vi "Big_LED_control.vi"() -> ()   [LabVIEW 2018]
uses:
  <instrlib>/niDCPower/nidcpower.llb/niDCPower Source Mode.ctl
  <instrlib>/niDCPower/nidcpower.llb/niDCPower Output Function.ctl
  AT lib/AmateurStepperMotor.dll
  <instrlib>/niDMM/nidmm.llb/niDMM Function.ctl
  <instrlib>/niDMM/nidmm.llb/niDMM Resolution in Digits.ctl
  <vilib>/Instr/_visa.llb/VISA Configure Serial Port (Instr).vi
  <instrlib>/niDMM/nidmm.llb/niDMM Configure Measurement Digits.vi
panel:
  out "Voltage Char 2":dbl(graph)=0.2558511793613434
  in  "Tab Control 2":enum32{"Шаговик и офир", "Служебная область"}(tab)
  in  "Go To":dbl
  out "Ophir 1 Char":dbl(graph)=0.02
  in  "DecelerationTime, s":dbl=0.3
  in  "AccelerationTime, s":dbl=0.3
  in  "HoldOn":bool
  in  "Ophir 1 units":string(combo)="1000" caption="Units"
  out "Ophir 1 Optical Power":dbl=0.02 caption="Power" format="%#_4g"
  out "Ophir 1 MAX":dbl=0.02 caption="MAX" format="%#_5g"
  in  "Ophir 1 Clear":bool caption="Clear"
  in  "StepMultiplicationFactor":dbl=50.0
  in  "StepDivisor":i32(ring)=8 items=["D1"=1, "D2"=2, "D4"=4, "D8"=8, "D16"=16, "D32"=32]
  in  "Speed":dbl=250.0
  in  "Погнали!":bool
  in  "Стоп GoTo":bool
  out "Готово":bool
  out "Position":dbl=9.995
  in  "Ophir 1 Info":u16(ring)=1 caption="Info" items=["Device : JUNO; s/n:903793", "Head : PD300R-3W   ; s/n:779628"]
  in  "new pos":dbl
  in  "set pos":bool
  in  "wave_lenght":string="600"
  in  "Ophir 1 usb channel":i16 caption="usb channel"
  out "Ophir 1 dup Visa Session":refnum<visa-resource-name>="USB0::0x0BD3::0x0777::NI-VISA-60003::RAW" caption="dup Visa Session"
  in  "Ophir 1 Baud Rate (3:9600)":i16(ring)=3 caption="Baud Rate (3:9600)" items=["300", "1200", "4800", "9600", "19200", "38400"]
  out "Ophir 1 Real Optical Power":dbl=2e-05 format="%.6e"
  in  "Ophir 1 GPIB Address (10)":string="10" caption="GPIB Address (10)"
  in  "Ophir 1 Port Number (default 2)":i16=1 caption="Port Number (default 2)" min=0 max=20
  in  "Ophir 1 Select Communication Protocol":u16(ring) caption="Select Communication Protocol" items=["USB", "RS232", "GPIB"]
  out "Ophir 1 error out":errorcluster caption="error out"
  in  "Ophir 1 error in (no error)":errorcluster caption="error in (no error)"
  in  "Ophir 1 Wait":u32=100 caption="Wait"
  out "IsOpen":bool
  out "Ophir 1 Initialization":bool=TRUE caption="Initialization"
  out "Device Response":string="*\n"
  in  "Tab Control":T1(tab)
  in  "шаговик":refnum<visa-resource-name>="COM8"
  in  "POWER":bool
  in  "Стоп":bool
  in  "Resource Name":refnum<k15>="PXI1Slot2" caption="Источник питания"
  in  "Амперметр":refnum<k15>="PXI1Slot4" caption="NI DMM 1"
  in  "V_MB, V":dbl=6.0 caption="voltage level" min=0.0 max=6.0 format="%_6p"
  in  "curlim_V_MB, A":dbl=0.3 caption="current limit" format="%_6p"
  out "chart_0":dbl(graph)=-0.00013853853853977013 caption="Waveform Chart 5"
  in  "voltlim_I_LED, V":dbl=2.1 caption="current limit" min=0.01 format="%_6p"
  in  "I_LED, A":dbl=0.010000000000000004 caption="voltage level" format="%_6p"
  out "chart_1":dbl(graph)=-0.0002744397184121777 caption="Waveform Chart 5"
  out "Current Char":dbl(graph)=0.0055655837059021
  in  "Arduino":refnum<visa-resource-name>="COM16"
  in  "Сегменты":bool[](array[boolean])=[FALSE, FALSE, FALSE, FALSE, FALSE, FALSE, FALSE, FALSE, FALSE, FALSE, FALSE, FALSE, FALSE, FALSE, FALSE, FALSE, FALSE, FALSE]
  in  "Вольтметр":refnum<k15>="PXI1Slot5" caption="NI DMM 1"
  out "Voltage Char":dbl(graph)=0.2558511793613434
  in  "Промер":bool caption="Промер сегмента"
  in  "NI DMM 1 Voltage Range 4":string(combo)="-1" caption="Range"
  in  "NI DMM 1 units 4":string(combo)="1" caption="Units"
  out "Voltage":dbl=0.2558511793613434 format="%_6g"
  in  "NI DMM 1 Current Range 3":string(combo)="1" caption="Range"
  in  "NI DMM 1 units 3":string(combo)="1000" caption="Units"
  out "Current":dbl format="%_6g"
  out "voltmes_V_MB, V":dbl=-0.00013853853853977013 caption="measurement" format="%_6g"
  out "curmes_V_MB, A":dbl caption="measurement" format="%_6g"
  out "curmes_I_LED, A":dbl=9.117163901385412e-07 caption="measurement" format="%_6g"
  out "voltmes_I_LED, V":dbl caption="measurement" format="%_6g"
  out "Разряд":dbl
  out "+/-":bool
  out "Power off":bool
  in  "Command":string="Cathode"
  in  "Записать":bool
  out "measure output \nfile refnum":refnum<file>
  out "Voltage, V":dbl=0.2558511793613434 caption="Measurement" format="%.5f"
  out "Current, A":dbl=5.5655837059021e-06 caption="Measurement" format="%.5f"
  out "Тип индикатора":string="Cathode"
  out "chart_2":dbl(graph)=0.0007584113885058215
  in  "V_RES, V":dbl caption="voltage level" format="%_6p"
  out "curmes_V_RES, A":dbl caption="measurement" format="%_6g"
  in  "curlim_V_RES, A":dbl=0.1 caption="current limit" min=0.01 format="%_6p"
  in  "measure path":path=path "C:/Users/user/Desktop/МСП/LabVIEW/LED_CONTROL_big_LED_ophir_24.12.24_1/Logs"
  out "Enum":enum16{"Exit", "4", "Промер", "2", "1"}(ring)
  out "№ об-ца":dbl
  out "Темп-ра":dbl
  out "Сегмент":string="n"
  out "voltmes_V_RES, V":dbl=0.0007584113885058215 caption="measurement" format="%_6g"
  in  "current level range":dbl=0.001 format="%#.6p"
  in  "range on/off":bool
  in  "I (np)":bool
  in  "II (Lm)":bool
  in  "III (jk)":bool
  in  "IV (gh)":bool
  in  "I - IV":bool
  # "Шаговик"
  # "Офир"
  # "Шаговик"
  # "Офир"
  # "position - это значение абсолютное"
  # "j"
  # "c"
  # "d"
  # "e"
  # "g"
  # "h"
  # "a"
  # "b"
  # "f"
  # "k"
  # "L"
  # "m"
  # "n"
  # "p"
  # "dp"
  # "all"
  # "1мА-30мА -> 1m\n10мА-1А -> off"
  # "V_MB 5 В\nогрничение 300 м\n\nV_LED 2,1 В\nограничение 200 м"
  # "единицы мА\nrange 1 А"
  # "1. каждый сегмент включаем по отдельности, резистором постраиваем ток до 10 мА\n2. напряжение V_LED при этом не меняется\n3. в такоом положении промеряем сегменты по отдельности\n4. для промера всего индикатора сразу подстраиваем напряжение при неизменном положении резисторов\n5. ток всех индикаторов = ток одного сегмента (10 мА) * число сегментов (15)\n6. добиваемся этого увеличением V_LED"
  # "единицы В\nrange AUTO"
  # "регклировка суммарного тока через индикатор"
  # "24.063\n\n     I          U\n20 мА  1.3 В\n20 мА  1.4 В\n 7 мА   1.15 В"
  # "24.064\n\n     I          U\n10 мА  2 В\n10 мА  2.15 В\n 7 мА   1.9 В"
  # "автоматизировать подбор напряжения по известному максимальному напряжению и току. ОС по току сегмента"
  # "Р1:  +25°C\nР2:  - 60°C\nР3:  +85°C"
  # "24.067 (в работе)"
  # "регулировать ток в зависимости от температуры.\nс ростом температуры растет ток.\nпид-регулятор??"
  # "0. ввести номер образца\n1. включить нужный сегмент\n2. ввести его в поле справа\n3. вести температуру в поле слева\n4. нажать кнопку \"промер сегмента\""
  # "\"опрашивать кнопки не чаще, чем раз в секунду. сейчас кликать можно чаще, они загорятся, но ничего не произойдет\""
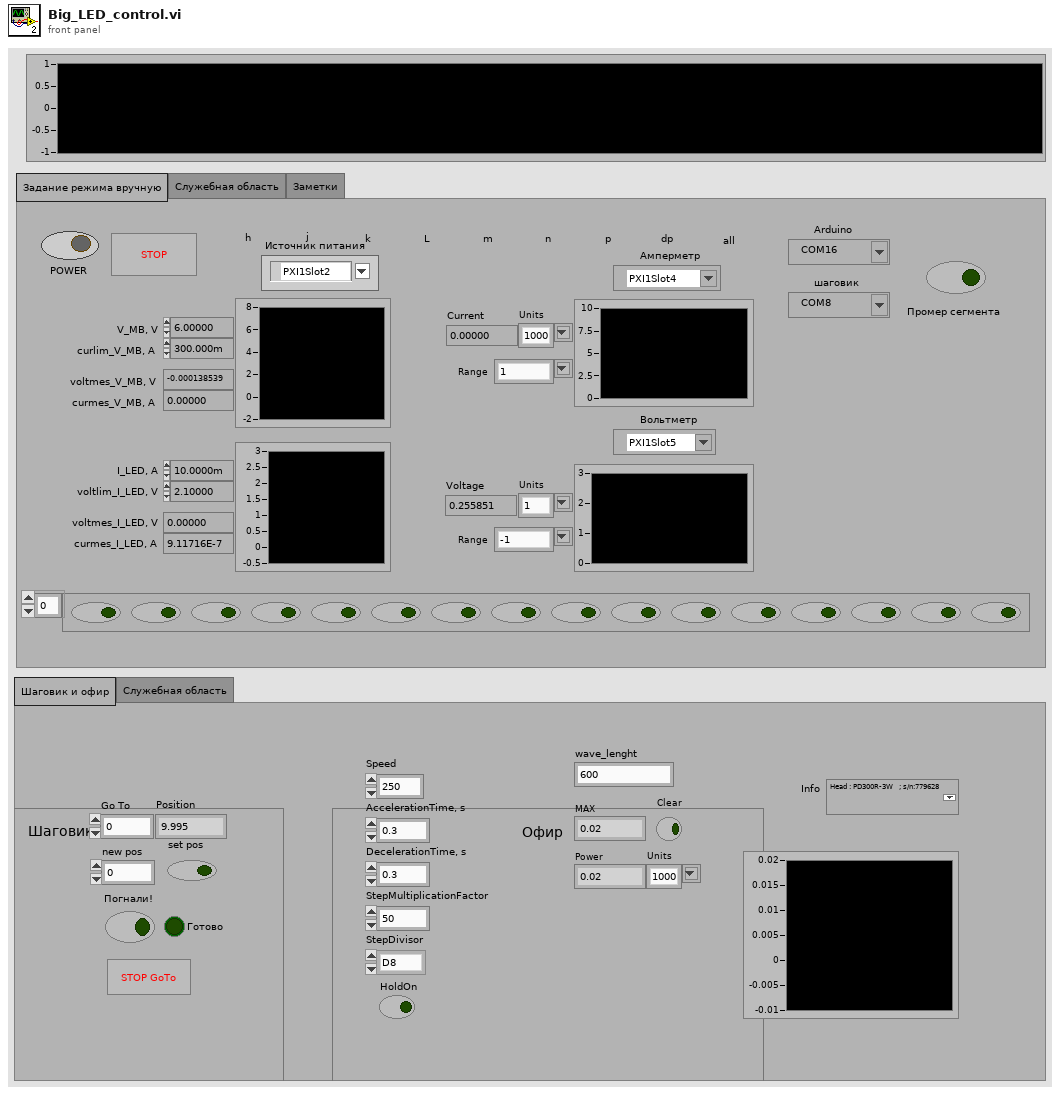
[diagram p1: front panel]
types:
  T1 = enum32{"Задание режима вручную", "Служебная область", "Заметки"}
  T2 = enum16{"open", "replace", "create", "open or create", "replace or create", "replace or create with confirmation"}
  T3 = typedef "niDCPower Output Function.ctl" = i32
  T4 = typedef "niDCPower Source Mode.ctl" = i32
  T5 = typedef "niDMM Function.ctl" = enum16{"DC Volts", "AC Volts", "DC Current", "AC Current", "2-wire Resistance", "4-wire Resistance", "Diode", "Frequency", "Period", "AC Volts DC Coupled", "Capacitance", "Inductance", "Temperature"}
  T6 = typedef "niDMM Resolution in Digits.ctl" = dbl
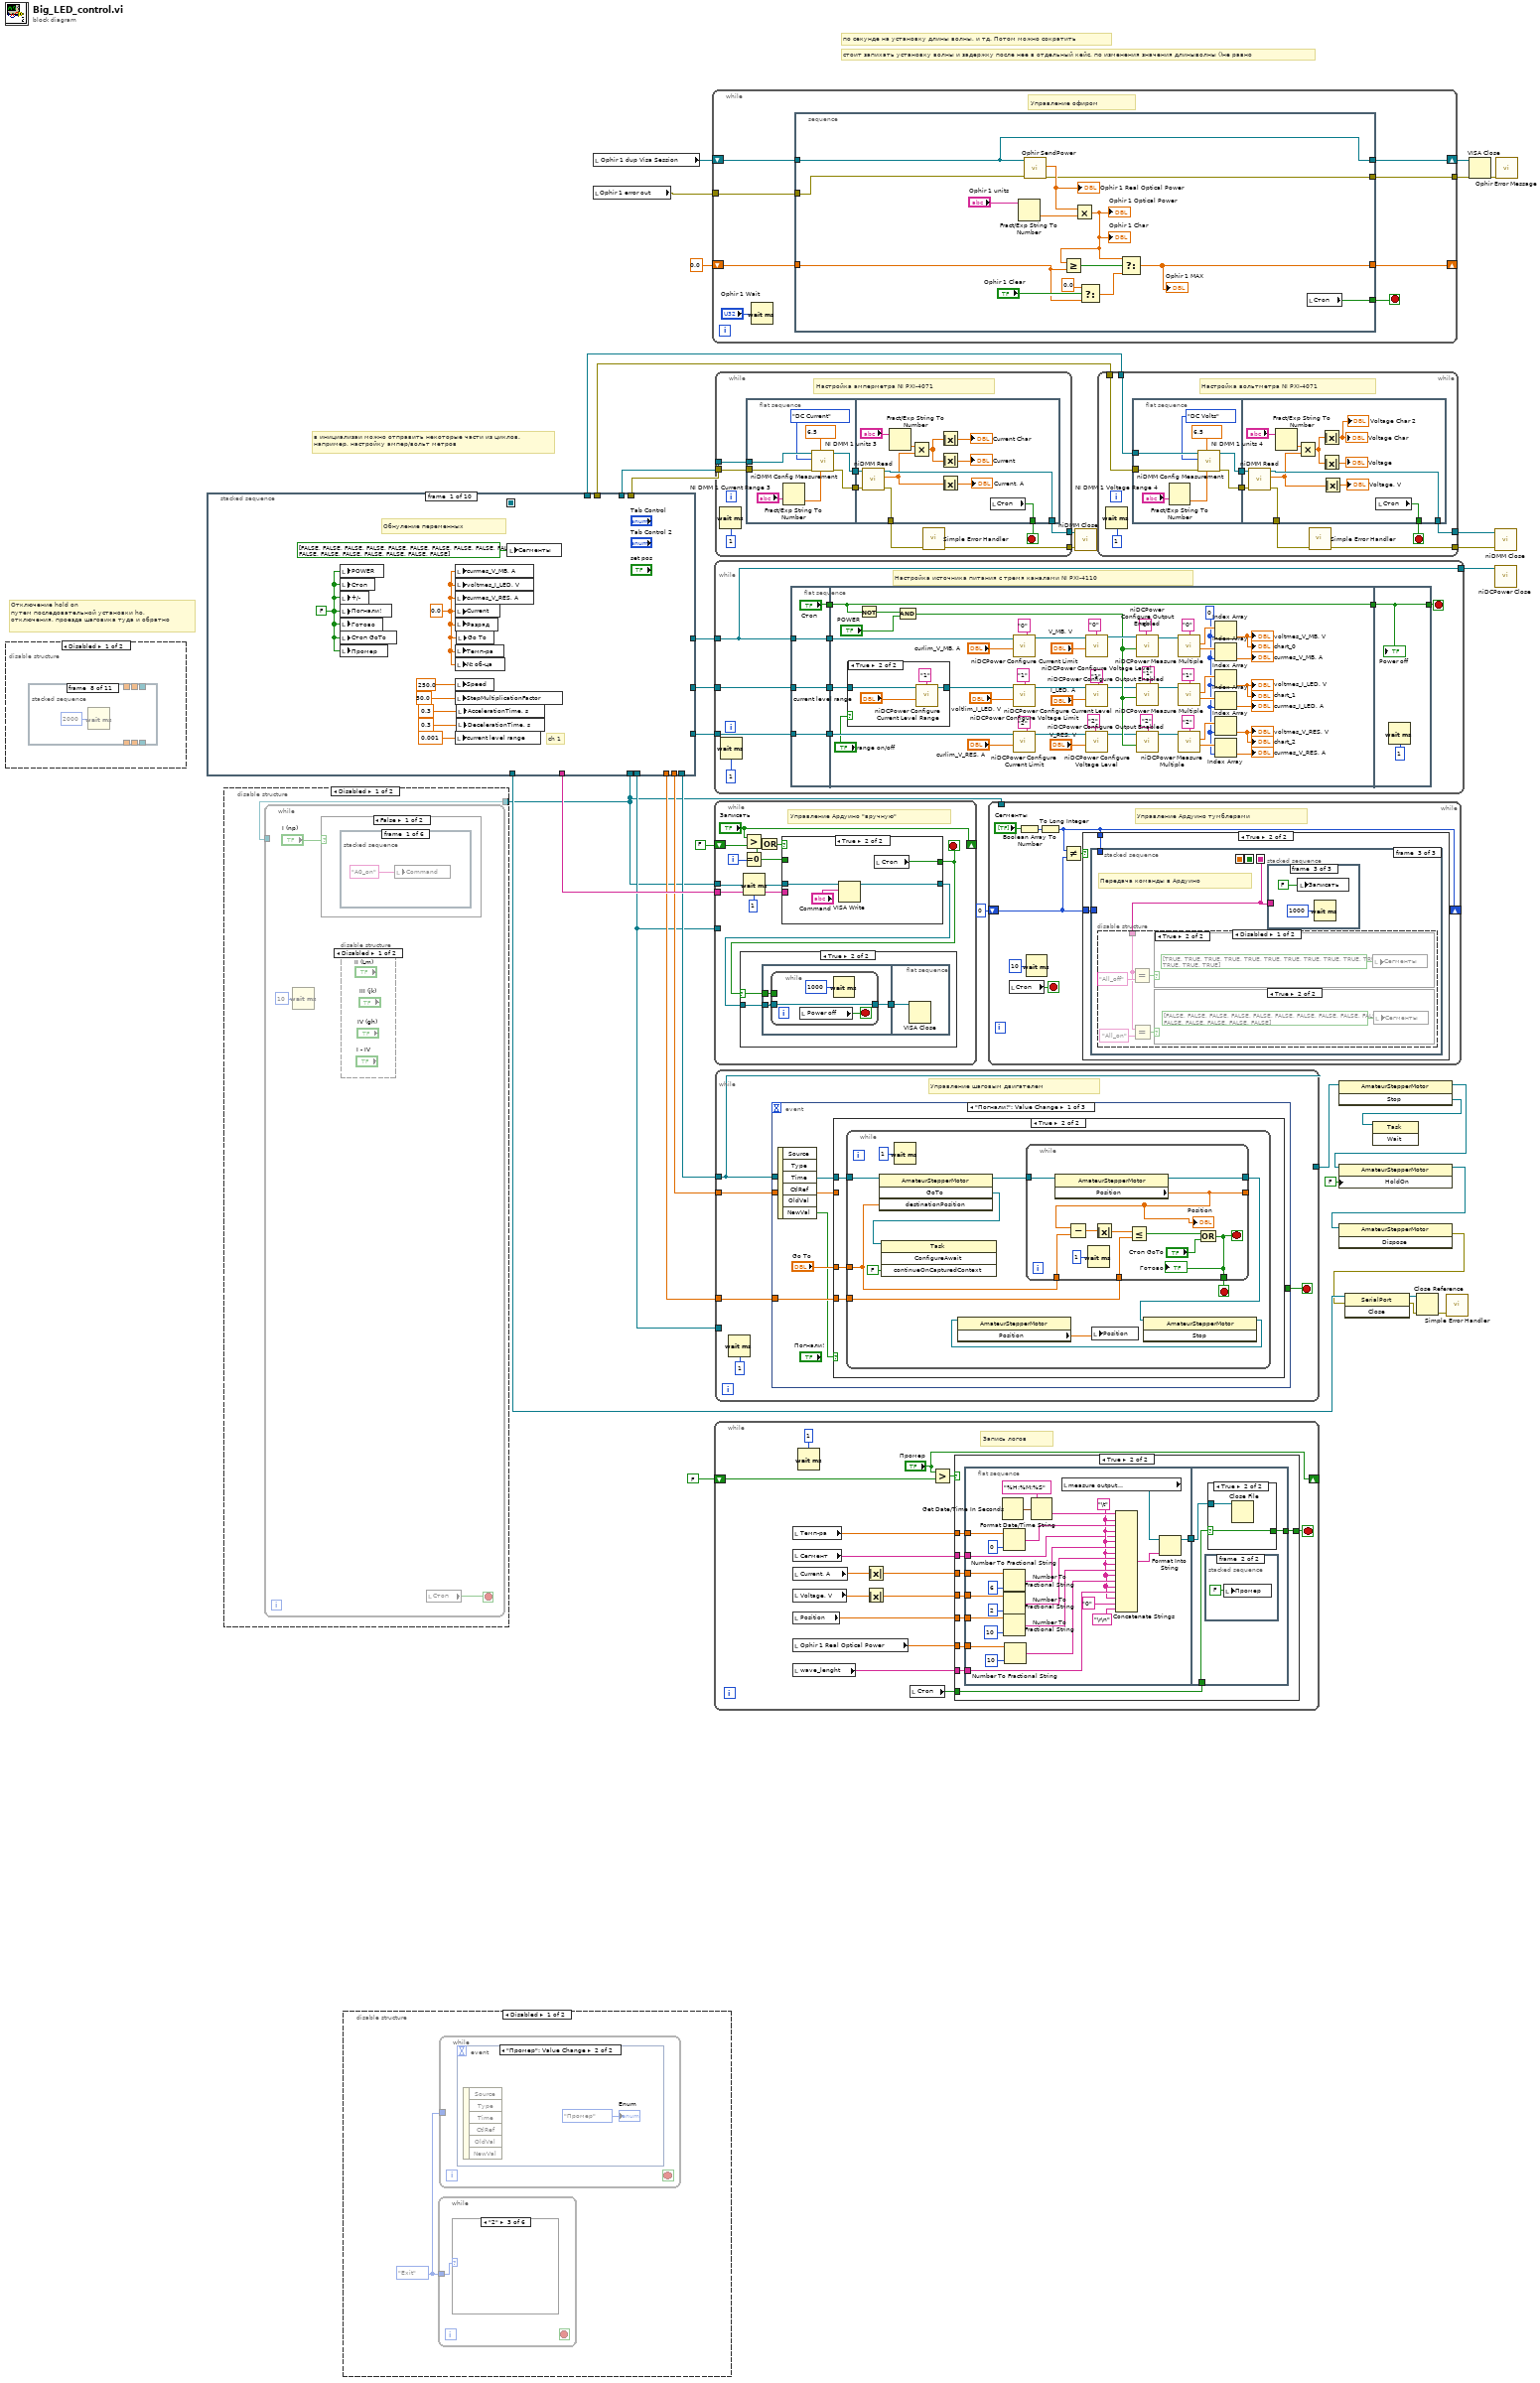
[diagram p0: block diagram]
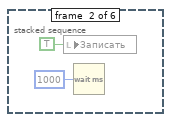
[diagram p3: hidden frame]
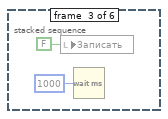
[diagram p4: hidden frame]
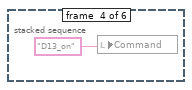
[diagram p5: hidden frame]
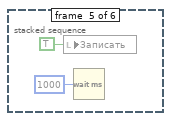
[diagram p6: hidden frame]
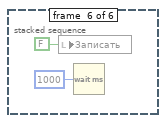
[diagram p7: hidden frame]
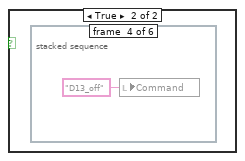
[diagram p8: hidden frame]
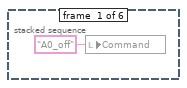
[diagram p9: hidden frame]
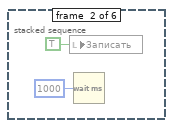
[diagram p10: hidden frame]
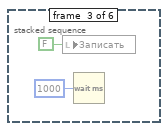
[diagram p11: hidden frame]
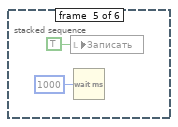
[diagram p12: hidden frame]
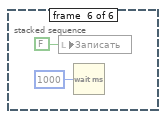
[diagram p13: hidden frame]
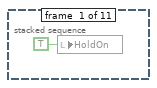
[diagram p15: hidden frame]
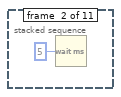
[diagram p16: hidden frame]
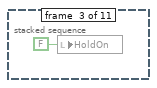
[diagram p17: hidden frame]
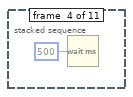
[diagram p18: hidden frame]
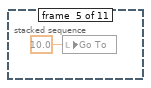
[diagram p19: hidden frame]
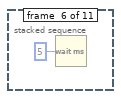
[diagram p20: hidden frame]
diagram:
  # "Отключение hold on\nпутем последовательной установки ho, \nотключения, проезда шаговика туда и обратно"
  # "в инициализаи можно отправить некоторые части из циклов.\nнапример, настройку ампер/вольт метров"
  # "стоит запихать установку волны и задержку после нее в отдельный кейс, по изменения значения длиныволны ()не равно"
  # "по секунде на установку длины волны, и тд. Потом можно сократить"
  n1 = disable-structure shown="Disabled" {
    frame Disabled {
      n2 = stacked-sequence {
        tunnel: _ -> [_ _ _ _ _ _ _ _ _ _ w50]
        tunnel: [_ _ _ _ _ _ _ _ _ _ w50] -> _
        tunnel: _ -> [_ _ _ _ _ _ _ _ _ _ w49]
        tunnel: [_ _ _ _ _ _ _ _ _ _ w49] -> _
        tunnel: [_ _ _ _ _ _ _ _ _ _ w48] -> _
        tunnel: _ -> [_ _ _ _ _ _ _ _ _ _ w48]
        frame #0 {
          n3 = local write "HoldOn"(TRUE ("HoldOn")) -> ()
        }
        frame #1 {
          n4 = Wait (ms)(milliseconds to wait=u32 5) -> ()  [unwired: 1 out]
        }
        frame #2 {
          n5 = local write "HoldOn"(FALSE ("HoldOn")) -> ()
        }
        frame #3 {
          n6 = Wait (ms)(milliseconds to wait=u32 500) -> ()  [unwired: 1 out]
        }
        frame #4 {
          n7 = local write "Go To"(10.0 ("Go To")) -> ()
        }
        frame #5 {
          n8 = Wait (ms)(milliseconds to wait=u32 5) -> ()  [unwired: 1 out]
        }
        frame #6 {
          n9 = local write "Погнали!"(TRUE ("Погнали!")) -> ()
        }
        frame #7 {
          n10 = Wait (ms)(milliseconds to wait=u32 2000) -> ()  [unwired: 1 out]
        }
        frame #8 {
          n11 = local write "Go To"(0.0 ("Go To")) -> ()
        }
        frame #9 {
          n12 = Wait (ms)(milliseconds to wait=u32 5) -> ()  [unwired: 1 out]
        }
        frame #10 {
          n13 = local write "Погнали!"(TRUE ("Погнали!")) -> ()
        }
      }
    }
    frame Enabled {
    }
  }
  n14 = stacked-sequence {
    seq-local: [_ _ _ _ _ _ w117 _ _ _] -> [_ _ _ _ _ _ _ w142 _ _]
    tunnel: [_ _ _ w68 _ _ _ _ _ _] -> w26
    tunnel: [_ w62 _ _ _ _ _ _ _ _] -> w37
    tunnel: [_ w61 _ _ _ _ _ _ _ _] -> w36
    tunnel: [_ _ _ _ w88 _ _ _ _ _] -> w1
    tunnel: [_ _ _ _ _ _ _ _ w148 _] -> w33
    tunnel: [_ _ w65 _ _ _ _ _ _ _] -> w32
    tunnel: [_ _ w64 _ _ _ _ _ _ _] -> w31
    tunnel: [_ _ _ _ _ _ _ w145 _ _] -> w3
    tunnel: [_ _ _ _ _ _ _ w143 _ _] -> w4
    tunnel: [_ _ _ _ _ _ _ w144 _ _] -> w5
    tunnel: [_ _ _ _ _ _ w119 _ _ _] -> w20
    tunnel: [_ _ _ w67 _ _ _ _ _ _] -> w8
    tunnel: [_ _ _ w66 _ _ _ _ _ _] -> w6
    tunnel: [_ _ _ _ _ _ _ _ _ w149] -> w2
    frame #0 {
      w52 = 0.0 ("currentmes_2")
      w53 = FALSE ("Стоп")
      # "ch 1"
      # "Обнуление переменных"
      n15 = local write "POWER"(w53) -> ()
      n16 = local write "Стоп"(w53) -> ()
      n17 = local write "+/-"(w53) -> ()
      n18 = local write "Погнали!"(w53) -> ()
      n19 = local write "Готово"(w53) -> ()
      n20 = local write "Стоп GoTo"(w53) -> ()
      n21 = local write "Промер"(w53) -> ()
      n22 = local write "curmes_V_MB, A"(w52) -> ()
      n23 = local write "voltmes_I_LED, V"(w52) -> ()
      n24 = local write "curmes_V_RES, A"(w52) -> ()
      n25 = local write "Current"(w52) -> ()
      n26 = local write "Разряд"(w52) -> ()
      n27 = local write "Темп-ра"(w52) -> ()
      n28 = local write "№ об-ца"(w52) -> ()
      n29 = local write "Speed"(250.0 ("Speed")) -> ()
      n30 = local write "StepMultiplicationFactor"(50.0 ("StepMultiplicationFactor")) -> ()
      n31 = local write "current level range"(0.001 ("current level range")) -> ()
      n32 = local write "Go To"(w52) -> ()
      n33 = local write "AccelerationTime, s"(0.3 ("AccelerationTime, s")) -> ()
      n34 = local write "DecelerationTime, s"(0.3 ("DecelerationTime, s")) -> ()
      n35 = local write "Сегменты"(bool[] [FALSE, FALSE, FALSE, FALSE, FALSE, FALSE, FALSE, FALSE, FALSE, FALSE, FALSE, FALSE, FALSE, FALSE, FALSE, FALSE, FALSE, FALSE] ("Сегменты")) -> ()
    }
    frame #1 {
      # "Инициализация амперметра"
      n36 = call <instrlib>:"niDMM Initialize.vi"("Instrument Descriptor"="Амперметр") -> ("error out"=w62:errorcluster, "instrument handle out"=w61:refnum<k15>)  [unwired: 9 in]
    }
    frame #2 {
      # "Инициализация вольтметра"
      n37 = call <instrlib>:"niDMM Initialize.vi"("Instrument Descriptor"="Вольтметр") -> ("error out"=w64:errorcluster, "instrument handle out"=w65:refnum<k15>)  [unwired: 9 in]
    }
    frame #3 {
      w73 = T3 1006 items=["DC Voltage"=1006, "DC Current"=1007, "Pulse Voltage"=1049, "Pulse Current"=1050] ("output function")
      w77 = T3 1007 items=["DC Voltage"=1006, "DC Current"=1007, "Pulse Voltage"=1049, "Pulse Current"=1050] ("output function")
      w78 = T3 1006 items=["DC Voltage"=1006, "DC Current"=1007, "Pulse Voltage"=1049, "Pulse Current"=1050] ("output function")
      w81 = T4 1020 items=["Single Point"=1020, "Sequence"=1021] ("source mode")
      # "Инициализация источника питания"
      n38 = call <instrlib>:"niDCPower Initialize.vi"("resource name"="Resource Name") -> ("instrument handle out"=w82:refnum<k15>)  [unwired: 3 in, 7 out]
      n39 = call <instrlib>:"niDCPower Configure Source Mode.vi"("source mode"=w81, "instrument handle"=w82) -> ("instrument handle out"=w72:refnum<k15>)  [unwired: 1 in, 8 out]
      n40 = call <instrlib>:"niDCPower Configure Output Function.vi"("output function"=w77, "channel name"="1", "instrument handle"=w72) -> ("instrument handle out"=w79:refnum<k15>)  [unwired: 7 in, 1 out]
      n41 = call <instrlib>:"niDCPower Configure Output Function.vi"("output function"=w73, "channel name"="2", "instrument handle"=w72) -> ("instrument handle out"=w74:refnum<k15>)  [unwired: 7 in, 1 out]
      n42 = call <instrlib>:"niDCPower Configure Output Function.vi"("output function"=w78, "channel name"="0", "instrument handle"=w72) -> ("instrument handle out"=w80:refnum<k15>)  [unwired: 7 in, 1 out]
      n43 = call <instrlib>:"niDCPower Configure Voltage Level.vi"("voltage level"=0.0, "channel name"="2", "instrument handle"=w74) -> ("instrument handle out"=w66:refnum<k15>)  [unwired: 7 in, 1 out]
      n44 = call <instrlib>:"niDCPower Configure Voltage Level.vi"("voltage level"=0.0, "channel name"="0", "instrument handle"=w80) -> ("instrument handle out"=w68:refnum<k15>)  [unwired: 7 in, 1 out]
      n45 = call <instrlib>:"niDCPower Configure Current Level.vi"("current level"=0.01, "channel name"="1", "instrument handle"=w79) -> ("instrument handle out"=w67:refnum<k15>)  [unwired: 7 in, 1 out]
    }
    frame #4 {
      # "Инициализация Ардуино"
      n46 = call-poly "VISA Configure Serial Port"("VISA resource name"="Arduino", "baud rate (9600)"=u32 9600) -> ("VISA resource name out"=w88:refnum<visa-resource-name>)  [unwired: 12 in, 1 out]
    }
    frame #5 {
      # "Инициализация офира"
      n47 = stacked-sequence {
        frame #0 {
          n48 = call "Ophir InitCom.vi"("GPIB Address (default 10)"="Ophir 1 GPIB Address (10)", "Communication (default USB 0)"="Ophir 1 Select Communication Protocol", "USB Channel number (default 0)"="Ophir 1 usb channel", "Port Number (default 2)"="Ophir 1 Port Number (default 2)", "error in (no error)"="Ophir 1 error in (no error)", "Baud Rate (3:9600)"="Ophir 1 Baud Rate (3:9600)") -> ("dup Visa Session"=w97:refnum<visa-resource-name>, "error out"=w96:errorcluster)  [unwired: 1 out]
          n49 = call "Ophir InstrInfo.vi"("Visa Session"=w97, "error in (no error)"=w96) -> ("dup Visa Session"=w109:refnum<visa-resource-name>, "Instrument Info"=w91:string, "error out"=w107:errorcluster)
          n50 = call "Ophir HeadInfo.vi"("Visa Session"=w109, "error in (no error)"=w107) -> ("error out"=w106:errorcluster, "dup Visa Session"=w108:refnum<visa-resource-name>, "Head Info"=w105:string)  [unwired: 6 out]
          n51 = call "Ophir InfoStrings.vi"("error in (no error)"=w106, "Head Info"=w105, "Instrument Info"=w91) -> ("error out"=w104:errorcluster, "Strings Array"=w103:string[])
          n52 = property on="Ophir 1 Info" class="Ring (strict)"("Strings []"=w103) -> ()  [unwired: 2 in, 2 out]
          n53 = call "Ophir ConfigDevice.vi"("Visa Session"=w108, "Measure Choice (0:Power)"=u16 0, "error in (no error)"=w104) -> ("dup Visa Session"=→"Ophir 1 dup Visa Session":refnum<visa-resource-name>, "OK ?"=→"Ophir 1 Initialization":bool, "error out"=→"Ophir 1 error out":errorcluster)  [unwired: 1 out]
        }
        frame #1 {
          n54 = local read "Ophir 1 dup Visa Session"() -> (w111:refnum<visa-resource-name>)
          n55 = local read "Ophir 1 error out"() -> (w112:errorcluster)
          n56 = call "light_setWaveLenght.vi"("error in (no error)"=w112, "Visa Session"=w111, "wave_lenght"="wave_lenght") -> ("Device Response"=→"Device Response":string)  [unwired: 6 in, 2 out]
        }
      }
    }
    frame #6 {
      w124 = 100 ("WriteTimeout")
      w128 = 1 items=["None", "One", "Two", "OnePointFive"] ("stopBits")
      w126 = 0 items=["None", "Odd", "Even", "Mark", "Space"] ("parity")
      # "убрали открытие порта. шаговик его и так сам откроет"
      # "Инициализация шаговика ч.1"
      n57 = constructor class="SerialPort"("portName"="шаговик", "baudRate"=57600, "parity"=w126, "dataBits"=8, "stopBits"=w128) -> (reference out=w123:refnum<k24>, error out=w122:errorcluster)  [unwired: 3 in, 6 out]
      n58 = property class="SerialPort"(reference=w123, error in=w122, "WriteTimeout"=w124, "ReadTimeout"=w124) -> (reference out=w119:refnum<k24>)  [unwired: 1 out]
      n59 = flat-sequence {
        tunnel: w119 -> [w135]
        tunnel: w118 -> [_]
        frame #0 {
          n60 = property class="SerialPort"(reference=w135) -> ("IsOpen"=→"IsOpen":bool)  [unwired: 1 in, 2 out]
        }
      }
      n61 = constructor class="AmateurStepperMotor"("serialPort"=w119) -> (reference out=w116:refnum<k24>, error out=w115:errorcluster)  [unwired: 3 in, 2 out]
      n62 = Not A Number/Path/Refnum?(number/path/refnum=w116) -> (NaN/Path/Refnum?=w120:bool)
      n63 = case shown="False" w120 {
        tunnel: w119 -> [_ w133]
        tunnel: [w129 w132] -> w118
        tunnel: [w130 w131] -> w117
        tunnel: w116 -> [w130 _]
        tunnel: w115 -> [w129 _]
        frame False {
        }
        frame True {
          n64 = constructor class="AmateurStepperMotor"("serialPort"=w133) -> (reference out=w131:refnum<k24>, error out=w132:errorcluster)  [unwired: 3 in, 2 out]
        }
      }
    }
    frame #7 {
      # "стоит допустить изменение\nтих параметров в цикле, а не только \nпри инициализации"
      # "это те самые 50 шагов за мм"
      # "Инициализация шаговика ч.2"
      n65 = property class="AmateurStepperMotor"(reference=w142, "Speed"="Speed", "StepDivisor"="StepDivisor", "StepMultiplicationFactor"="StepMultiplicationFactor", "AccelerationTime"="AccelerationTime, s", "DecelerationTime"="DecelerationTime, s", "HoldOn"="HoldOn") -> (reference out=w145:refnum<k24>, "Position"=w143:dbl, "PositioningPrecision"=w144:dbl)  [unwired: 1 in, 1 out]
    }
    frame #8 {
      # "Begin VI: ОК или ОА?"
      n66 = call "Begin.vi"() -> ("Темп-ра"=→"Темп-ра":dbl, "№ об-ца"=→"№ об-ца":dbl, "String"=w148:string)  [unwired: 6 in]
      "Тип индикатора" <- w148
      n67 = local write "Command"(w148) -> ()
    }
    frame #9 {
      w159 = "\t"
      # "Инициализация логов"
      n68 = local read "№ об-ца"() -> (w163:dbl)
      n69 = Number To Fractional String(number=w163, precision (6)=i16 0) -> (F-format string=w164:string)  [unwired: 2 in]
      n70 = Get Date/Time In Seconds() -> (seconds since 1Jan1904=w174:timestamp)
      n71 = Build Path(base path="measure path", name or relative path=w164) -> (appended path=w170:path)
      n72 = call <vilib>:"Check if File or Folder Exists.vi"("path"=w170) -> ("file or folder exists?"=w171:bool, "dup path"=w172:path)  [unwired: 8 in, 1 out]
      n73 = Format Date/Time String(time format string (%c)="MES %d. %m. %y %H.%M.%S", seconds (now)=w174) -> (date/time string=w175:string)  [unwired: 1 in]
      n74 = case shown="True" w171 {
        tunnel: w172 -> [w181 w182]
        tunnel: [w180 w182] -> w173
        frame False {
          n75 = Create Folder(path (use dialog)=w181) -> (created path=w180:path)  [unwired: 2 in, 2 out]
        }
        frame True {
        }
      }
      n76 = Concatenate Strings(w175, ".xls" ("string")) -> (w176:string)
      n77 = Build Path(base path=w173, name or relative path=w176) -> (appended path=w177:path)
      n78 = Open/Create/Replace File(file path (use dialog)=w177, operation (0:open)=T2."open or create", access (0:read/write)=enum16{"read/write", "read-only", "write-only"}."read/write") -> (refnum out=w178:refnum<file>)  [unwired: 3 in, 2 out]
      n79 = Set File Position(refnum=w178, from (0:start)=enum16{"start", "end", "current"}."end") -> (refnum out=w161:refnum<file>)  [unwired: 2 in, 1 out]
      n80 = Format Into String(initial string=w161, "Time" ("string"), w159, "Temperature, C" ("string"), w159, "Segment" ("string"), w159, "Current, mA" ("string"), w159, "Voltage, V" ("input 7"), w159, "Distance, m" ("string"), w159, "Power, W " ("string"), w159, "Wavelenght, nm" ("input 17"), w159, "Candlepower, kd" ("string"), "\r\n") -> (resulting string=w149:refnum<file>)  [unwired: 2 in, 1 out]
      "measure output \nfile refnum" <- w149
    }
  }
  n81 = disable-structure shown="Disabled" {
    disable-tunnel: w1 -> [w183 _]
    frame Disabled {
      n82 = while {
        tunnel: w183 -> [_]
        stop <- w185 stop-if-true
        n83 = Wait (ms)(milliseconds to wait=u32 10 ("millisecond timer value")) -> ()  [unwired: 1 out]
        n84 = case shown="False" "I (np)" {
          frame False {
            n85 = stacked-sequence {
              frame #0 {
                n86 = local write "Command"("A0_on" ("Command")) -> ()
              }
              frame #1 {
                n87 = local write "Записать"(TRUE ("Записать")) -> ()
                n88 = Wait (ms)(milliseconds to wait=u32 1000) -> ()  [unwired: 1 out]
              }
              frame #2 {
                n89 = local write "Записать"(FALSE ("Записать")) -> ()
                n90 = Wait (ms)(milliseconds to wait=u32 1000) -> ()  [unwired: 1 out]
              }
              frame #3 {
                n91 = local write "Command"("D13_on" ("Command")) -> ()
              }
              frame #4 {
                n92 = local write "Записать"(TRUE ("Записать")) -> ()
                n93 = Wait (ms)(milliseconds to wait=u32 1000) -> ()  [unwired: 1 out]
              }
              frame #5 {
                n94 = local write "Записать"(FALSE ("Записать")) -> ()
                n95 = Wait (ms)(milliseconds to wait=u32 1000) -> ()  [unwired: 1 out]
              }
            }
          }
          frame True {
            n96 = stacked-sequence {
              frame #0 {
                n97 = local write "Command"("A0_off" ("Command")) -> ()
              }
              frame #1 {
                n98 = local write "Записать"(TRUE ("Записать")) -> ()
                n99 = Wait (ms)(milliseconds to wait=u32 1000) -> ()  [unwired: 1 out]
              }
              frame #2 {
                n100 = local write "Записать"(FALSE ("Записать")) -> ()
                n101 = Wait (ms)(milliseconds to wait=u32 1000) -> ()  [unwired: 1 out]
              }
              frame #3 {
                n102 = local write "Command"("D13_off" ("Command")) -> ()
              }
              frame #4 {
                n103 = local write "Записать"(TRUE ("Записать")) -> ()
                n104 = Wait (ms)(milliseconds to wait=u32 1000) -> ()  [unwired: 1 out]
              }
              frame #5 {
                n105 = local write "Записать"(FALSE ("Записать")) -> ()
                n106 = Wait (ms)(milliseconds to wait=u32 1000) -> ()  [unwired: 1 out]
              }
            }
          }
        }
        n107 = disable-structure shown="Disabled" {
          frame Disabled {
          }
          frame Enabled {
          }
        }
        n108 = local read "Стоп"() -> (w185:bool)
      }
    }
    frame Enabled {
    }
  }
  n109 = disable-structure shown="Disabled" {
    frame Disabled {
      w207 = enum16{"Exit", "4", "Промер", "2", "1"}."Exit"
      n110 = while {
        tunnel: w207 -> [w208]
        stop <- _ stop-if-true
        n111 = case shown="\"2\"" w208 {
          frame "Exit", Default {
          }
          frame "4" {
          }
          frame "2" {
          }
          frame "2" {
          }
          frame "1" {
          }
          frame "Промер" {
          }
        }
      }
      n112 = while {
        tunnel: w207 -> [_]
        stop <- _ stop-if-true
        n113 = event shown="[1] \"Промер\": Value Change" {
          selector: _ -> [_ _]
          dyn-events: _ -> [_ _]
          timeout: _ -> [_ _]
          event Timeout {
            n114 = event-data() -> ()  [unwired: 1 in, 3 out]
          }
          event "Промер": Value Change {
            n115 = event-data() -> ()  [unwired: 1 in, 6 out]
            "Enum" <- enum16{"Exit", "4", "Промер", "2", "1"}."Промер" ("Enum")
          }
        }
      }
    }
    frame Enabled {
    }
  }
  n116 = local read "Ophir 1 error out"() -> (w24:errorcluster)
  n117 = local read "Ophir 1 dup Visa Session"() -> (w25:refnum<visa-resource-name>)
  n118 = while {
    tunnel: w24 -> [w216]
    shift-right: [w212] -> _
    shift-left: 0.0 ("t") -> [w215]
    shift-right: [w213] -> w18
    shift-left: w25 -> [w217]
    tunnel: [w211] -> w17
    stop <- w210 stop-if-true
    # "Управление офиром"
    n119 = Wait (ms)(milliseconds to wait="Ophir 1 Wait") -> ()  [unwired: 1 out]
    n120 = stacked-sequence {
      tunnel: w217 -> [w219]
      tunnel: w216 -> [w221]
      tunnel: w215 -> [w222]
      tunnel: [w219] -> w213
      tunnel: [w223] -> w212
      tunnel: [w220] -> w211
      tunnel: [w218] -> w210
      frame #0 {
        n121 = Fract/Exp String To Number(string="Ophir 1 units") -> (number=w226:dbl)  [unwired: 3 in, 1 out]
        n122 = call "Ophir SendPower.vi"("Visa Session"=w219, "error in (no error)"=w221) -> ("Value Number"=w225:dbl, "error out"=w220:errorcluster)  [unwired: 2 out]
        "Ophir 1 Real Optical Power" <- w225
        n123 = Multiply(x=w225, y=w226) -> (x*y=w229:dbl)
        "Ophir 1 Char" <- w229
        "Ophir 1 Optical Power" <- w229
        n124 = Greater Or Equal?(x=w229, y=w222) -> (x >= y?=w230:bool)
        n125 = Select(t=0.0, s="Ophir 1 Clear", f=w222) -> (s? t:f=w228:dbl)
        n126 = Select(t=w229, s=w230, f=w228) -> (s? t:f=w223:dbl)
        "Ophir 1 MAX" <- w223
        n127 = local read "Стоп"() -> (w218:bool)
      }
    }
  }
  n128 = while {
    tunnel: w26 -> [w238]
    tunnel: [w238] -> w34
    tunnel: w8 -> [w235]
    tunnel: w6 -> [w232]
    stop <- w234 stop-if-true
    # "Настройка источника питания с тремя каналами NI PXI-4110"
    n129 = Wait (ms)(milliseconds to wait=u32 1) -> ()  [unwired: 1 out]
    n130 = flat-sequence {
      tunnel: w238 -> [w245]
      tunnel: [w245] -> w240
      tunnel: ["Стоп"] -> w239
      tunnel: [w243] -> w236
      tunnel: w235 -> [w243]
      tunnel: [w242] -> w233
      tunnel: w232 -> [w242]
      tunnel: w240 -> [w290]
      tunnel: w239 -> [w294]
      tunnel: [w294] -> w237
      tunnel: w236 -> [w258]
      tunnel: w233 -> [w253]
      tunnel: [w301] -> w234
      tunnel: w237 -> [w301]
      frame #0 {
      }
      frame #1 {
        w259 = 0 ("index")
        n131 = case shown="True" "range on/off" {
          tunnel: w258 -> [w295 w299]
          tunnel: [w295 w298] -> w257
          frame False {
          }
          frame True {
            n132 = call <instrlib>:"niDCPower Configure Current Level Range.vi"("current level range"="current level range", "channel name"="1", "instrument handle"=w299) -> ("instrument handle out"=w298:refnum<k15>)  [unwired: 7 in, 1 out]
          }
        }
        n133 = Not(x=w294) -> (.not. x?=w293:bool)
        n134 = And(x=w293, y="POWER") -> (x .and. y?=w289:bool)
        n135 = call <instrlib>:"niDCPower Configure Current Limit.vi"("current limit"="curlim_V_MB, A", "channel name"="0", "instrument handle"=w290) -> ("instrument handle out"=w280:refnum<k15>)  [unwired: 7 in, 1 out]
        n136 = call <instrlib>:"niDCPower Configure Voltage Limit.vi"("voltage limit"="voltlim_I_LED, V", "channel name"="1", "instrument handle"=w257) -> ("instrument handle out"=w284:refnum<k15>)  [unwired: 7 in, 1 out]
        n137 = call <instrlib>:"niDCPower Configure Current Limit.vi"("current limit"="curlim_V_RES, A", "channel name"="2", "instrument handle"=w253) -> ("instrument handle out"=w274:refnum<k15>)  [unwired: 7 in, 1 out]
        n138 = call <instrlib>:"niDCPower Configure Voltage Level.vi"("voltage level"="V_MB, V", "channel name"="0", "instrument handle"=w280) -> ("instrument handle out"=w291:refnum<k15>)  [unwired: 7 in, 1 out]
        n139 = call <instrlib>:"niDCPower Configure Current Level.vi"("current level"="I_LED, A", "channel name"="1", "instrument handle"=w284) -> ("instrument handle out"=w285:refnum<k15>)  [unwired: 7 in, 1 out]
        n140 = call <instrlib>:"niDCPower Configure Voltage Level.vi"("voltage level"="V_RES, V", "channel name"="2", "instrument handle"=w274) -> ("instrument handle out"=w275:refnum<k15>)  [unwired: 7 in, 1 out]
        n141 = call <instrlib>:"niDCPower Configure Output Enabled.vi"("output enabled"=w289, "channel name"="0", "instrument handle"=w291) -> ("instrument handle out"=w268:refnum<k15>)  [unwired: 7 in, 1 out]
        n142 = call <instrlib>:"niDCPower Configure Output Enabled.vi"("output enabled"=w289, "channel name"="1", "instrument handle"=w285) -> ("instrument handle out"=w261:refnum<k15>)  [unwired: 7 in, 1 out]
        n143 = call <instrlib>:"niDCPower Configure Output Enabled.vi"("output enabled"=w289, "channel name"="2", "instrument handle"=w275) -> ("instrument handle out"=w260:refnum<k15>)  [unwired: 7 in, 1 out]
        n144 = call <instrlib>:"niDCPower Measure Multiple.vi"("channel name"="0", "instrument handle"=w268) -> ("current measurements"=w266:dbl[], "voltage measurements"=w267:dbl[])  [unwired: 6 in, 2 out]
        n145 = call <instrlib>:"niDCPower Measure Multiple.vi"("channel name"="1", "instrument handle"=w261) -> ("current measurements"=w264:dbl[], "voltage measurements"=w265:dbl[])  [unwired: 6 in, 2 out]
        n146 = call <instrlib>:"niDCPower Measure Multiple.vi"("channel name"="2", "instrument handle"=w260) -> ("current measurements"=w262:dbl[], "voltage measurements"=w263:dbl[])  [unwired: 6 in, 2 out]
        n147 = Index Array(array=w267, index=w259) -> (element=→"chart_0" →"voltmes_V_MB, V":dbl)
        n148 = Index Array(array=w266, index=w259) -> (element=→"curmes_V_MB, A":dbl)
        n149 = Index Array(array=w265, index=w259) -> (element=→"chart_1" →"voltmes_I_LED, V":dbl)
        n150 = Index Array(array=w264, index=w259) -> (element=→"curmes_I_LED, A":dbl)
        n151 = Index Array(array=w263, index=w259) -> (element=→"chart_2" →"voltmes_V_RES, V":dbl)
        n152 = Index Array(array=w262, index=w259) -> (element=→"curmes_V_RES, A":dbl)
      }
      frame #2 {
        n153 = Wait (ms)(milliseconds to wait=u32 1) -> ()  [unwired: 1 out]
        "Power off" <- w301
      }
    }
  }
  n154 = while {
    tunnel: w1 -> [w309]
    shift-right: ["Записать"] -> _
    shift-left: FALSE ("Записать") -> [w311]
    tunnel: w33 -> [w307]
    tunnel: w2 -> [_]
    i -> [w308]
    stop <- w302 stop-if-true
    # "Управление Ардуино \"вручную\""
    n155 = Greater?(x="Записать", y=w311) -> (0:w305:bool)
    n156 = Equal To 0?(x=w308) -> (x = 0?=w304:bool)
    n157 = Wait (ms)(milliseconds to wait=u32 1) -> ()  [unwired: 1 out]
    n158 = Or(x=w305, y=w304) -> (x .or. y?=w306:bool)
    n159 = case shown="True" w306 {
      tunnel: w309 -> [w323 w328]
      tunnel: [w324 w327] -> w302
      tunnel: w307 -> [_ _]
      tunnel: w304 -> [_ _]
      tunnel: [w323 w325] -> w303
      frame False {
        n160 = local read "Стоп"() -> (w324:bool)
      }
      frame True {
        n161 = VISA Write(VISA resource name=w328, write buffer="Command") -> (VISA resource name out=w325:refnum<visa-resource-name>)  [unwired: 1 in, 2 out]
        n162 = local read "Стоп"() -> (w327:bool)
      }
    }
    n163 = case shown="True" w302 {
      selector: w302 -> [_ w313]
      tunnel: w303 -> [_ w315]
      frame False {
      }
      frame True {
        n164 = flat-sequence {
          tunnel: w315 -> [w318]
          tunnel: [w317] -> w314
          tunnel: w313 -> [w316]
          tunnel: w314 -> [w322]
          frame #0 {
            n165 = while {
              tunnel: w318 -> [w321]
              tunnel: [w321] -> w317
              tunnel: w316 -> [_]
              stop <- w319 stop-if-true
              n166 = local read "Power off"() -> (w319:bool)
              n167 = Wait (ms)(milliseconds to wait=u32 1000) -> ()  [unwired: 1 out]
            }
          }
          frame #1 {
            n168 = VISA Close(VISA resource name=w322) -> ()  [unwired: 1 in, 1 out]
          }
        }
      }
    }
  }
  n169 = while {
    shift-right: ["Промер"] -> _
    shift-left: FALSE ("Промер сегмента") -> [w341]
    stop <- w338 stop-if-true
    # "Запиcь логов"
    n170 = local read "Темп-ра"() -> (w334:dbl)
    n171 = local read "Сегмент"() -> (w335:string)
    n172 = local read "Current, A"() -> (w337:dbl)
    n173 = local read "Voltage, V"() -> (w336:dbl)
    n174 = local read "Position"() -> (w333:dbl)
    n175 = local read "Ophir 1 Real Optical Power"() -> (w332:dbl)
    n176 = local read "wave_lenght"() -> (w329:string)
    n177 = Wait (ms)(milliseconds to wait=u32 1) -> ()  [unwired: 1 out]
    n178 = Absolute Value(x=w337) -> (abs(x)=w330:dbl)
    n179 = Absolute Value(x=w336) -> (abs(x)=w331:dbl)
    n180 = local read "Стоп"() -> (w339:bool)
    n181 = Greater?(x="Промер", y=w341) -> (0:w342:bool)
    n182 = case shown="True" w342 {
      tunnel: w330 -> [_ w354]
      tunnel: w331 -> [_ w353]
      tunnel: w333 -> [_ w350]
      tunnel: w332 -> [_ w351]
      tunnel: w329 -> [_ w352]
      tunnel: w339 -> [w344 w348]
      tunnel: w334 -> [_ w347]
      tunnel: w335 -> [_ w346]
      tunnel: [w344 w345] -> w338
      frame False {
      }
      frame True {
        n183 = flat-sequence {
          tunnel: w354 -> [w372]
          tunnel: w353 -> [w371]
          tunnel: w352 -> [w369]
          tunnel: w351 -> [w368]
          tunnel: w350 -> [w367]
          tunnel: [w362] -> w349
          tunnel: w347 -> [w361]
          tunnel: w346 -> [w355]
          tunnel: w349 -> [w383]
          tunnel: w348 -> [w382]
          tunnel: [w381] -> w345
          frame #0 {
            w357 = "\t"
            n184 = Get Date/Time In Seconds() -> (seconds since 1Jan1904=w380:timestamp)
            n185 = Number To Fractional String(number=w361, precision (6)=i16 0) -> (F-format string=w359:string)  [unwired: 2 in]
            n186 = Number To Fractional String(number=w372, precision (6)=i16 6) -> (F-format string=w375:string)  [unwired: 2 in]
            n187 = Number To Fractional String(number=w371, precision (6)=i16 2) -> (F-format string=w374:string)  [unwired: 2 in]
            n188 = Number To Fractional String(number=w367, precision (6)=i16 10) -> (F-format string=w373:string)  [unwired: 2 in]
            n189 = Number To Fractional String(number=w368, precision (6)=i16 10) -> (F-format string=w370:string)  [unwired: 2 in]
            n190 = Format Date/Time String(time format string (%c)="%H:%M:%S", seconds (now)=w380) -> (date/time string=w378:string)  [unwired: 1 in]
            n191 = local read "measure output \nfile refnum"() -> (w376:refnum<file>)
            n192 = Concatenate Strings(w378, w357, w359, w357, w355, w357, w375, w357, w374, w357, w373, w357, w370, w357, w369, w357, "0" ("string"), "\r\n") -> (w377:string)
            n193 = Format Into String(initial string=w376, w377) -> (resulting string=w362:refnum<file>)  [unwired: 2 in, 1 out]
          }
          frame #1 {
            n194 = stacked-sequence {
              frame #0 {
                n195 = Wait (ms)(milliseconds to wait=u32 250) -> ()  [unwired: 1 out]
              }
              frame #1 {
                n196 = local write "Промер"(FALSE ("Промер")) -> ()
              }
            }
            n197 = case shown="True" w382 {
              selector: w382 -> [_ w387]
              tunnel: w383 -> [_ w388]
              tunnel: [FALSE w387] -> w381
              frame False {
              }
              frame True {
                n198 = Close File(refnum=w388) -> ()  [unwired: 1 in, 2 out]
              }
            }
          }
        }
      }
    }
  }
  n199 = while {
    tunnel: [w395] -> w27
    tunnel: w36 -> [w393]
    tunnel: w37 -> [w392]
    tunnel: [w389] -> w28
    stop <- w391 stop-if-true
    # "Настройка амперметра NI PXI-4071"
    n200 = Wait (ms)(milliseconds to wait=u32 1) -> ()  [unwired: 1 out]
    n201 = flat-sequence {
      tunnel: [w402] -> w397
      tunnel: w393 -> [w400]
      tunnel: w392 -> [w404]
      tunnel: [w401] -> w396
      tunnel: w397 -> [w414]
      tunnel: w396 -> [w417]
      tunnel: [w413] -> w391
      tunnel: [w412] -> w389
      tunnel: [w411] -> w390
      frame #0 {
        w398 = T6 6.5 items=["3 1/2"=3.5, "4 1/2"=4.5, "5 1/2"=5.5, "6 1/2"=6.5, "7 1/2"=7.5] ("Resolution in Digits")
        n202 = Fract/Exp String To Number(string="NI DMM 1 Current Range 3") -> (number=w403:dbl)  [unwired: 3 in, 1 out]
        n203 = call-poly <instrlib>:"niDMM Config Measurement.vi"("Range"=w403, "Resolution in Digits"=w398, "error in (no error)"=w404, "Function"=niDMM_Function."DC Current" ("Measurement Type"), "instrument handle"=w400) -> ("error out"=w401:errorcluster, "instrument handle out"=w402:refnum<k15>)  [unwired: 5 in]
      }
      frame #1 {
        n204 = call <instrlib>:"niDMM Read.vi"("error in (no error)"=w417, "instrument handle"=w414) -> ("error out"=w411:errorcluster, "Measurement"=w406:dbl, "instrument handle out"=w412:refnum<k15>)  [unwired: 7 in]
        n205 = Fract/Exp String To Number(string="NI DMM 1 units 3") -> (number=w415:dbl)  [unwired: 3 in, 1 out]
        n206 = Multiply(x=w415, y=w406) -> (x*y=w408:dbl)
        n207 = Absolute Value(x=w408) -> (abs(x)=→"Current Char":dbl)
        n208 = Absolute Value(x=w408) -> (abs(x)=→"Current":dbl)
        n209 = Absolute Value(x=w406) -> (abs(x)=→"Current, A":dbl)
        n210 = local read "Стоп"() -> (w413:bool)
      }
    }
    n211 = call <vilib>:"Simple Error Handler.vi"("error in (no error)"=w390) -> ("error out"=w395:errorcluster)  [unwired: 1 in, 7 out]
  }
  n212 = while {
    tunnel: w3 -> [w419]
    tunnel: w5 -> [w421]
    tunnel: [w419] -> w7
    tunnel: w4 -> [w422]
    tunnel: w2 -> [_]
    stop <- w418 stop-if-true
    # "Управление шаговым двигателем"
    n213 = Wait (ms)(milliseconds to wait=u32 1) -> ()  [unwired: 1 out]
    n214 = event shown="[0] \"Погнали!\": Value Change" {
      selector: _ -> [_ _ _]
      dyn-events: _ -> [_ _ _]
      timeout: _ -> [_ _ _]
      tunnel: w419 -> [w427 w455 _]
      tunnel: w422 -> [w426 _ _]
      tunnel: w421 -> [w425 _ _]
      tunnel: [_ _ w461] -> w418
      event "Погнали!": Value Change {
        n215 = event-data() -> ("NewVal"=w423:bool)  [unwired: 1 in, 5 out]
        n216 = case shown="True" w423 {
          tunnel: "Go To" -> [_ w431]
          tunnel: w427 -> [_ w430]
          tunnel: w426 -> [_ _]
          tunnel: w425 -> [_ w429]
          frame False {
            n217 = Wait (ms)(milliseconds to wait=u32 1) -> ()  [unwired: 1 out]
          }
          frame True {
            n218 = while {
              tunnel: w431 -> [w438]
              tunnel: w430 -> [w439]
              tunnel: w429 -> [w441]
              stop <- w442 stop-if-true
              n219 = invoke class="AmateurStepperMotor" method="GoTo"(reference=w439, "destinationPosition"=w438) -> (reference out=w434:refnum<k24>, "GoTo"=w437:refnum<k24>)  [unwired: 2 in, 2 out]
              n220 = invoke class="Task" method="ConfigureAwait"(reference=w437, "continueOnCapturedContext"=FALSE) -> ()  [unwired: 2 in, 4 out]
              n221 = Wait (ms)(milliseconds to wait=u32 1) -> ()  [unwired: 1 out]
              n222 = while {
                tunnel: [w443] -> _
                tunnel: [w445] -> w435
                tunnel: [w447] -> w442
                tunnel: w438 -> [w452]
                tunnel: w441 -> [w450]
                tunnel: w434 -> [w444]
                stop <- w447 stop-if-true
                n223 = property class="AmateurStepperMotor"(reference=w444) -> (reference out=w445:refnum<k24>, "Position"=w443:dbl)  [unwired: 1 in, 1 out]
                "Position" <- w443
                n224 = Subtract(x=w443, y=w452) -> (x-y=w453:dbl)
                n225 = Wait (ms)(milliseconds to wait=u32 1) -> ()  [unwired: 1 out]
                n226 = Absolute Value(x=w453) -> (abs(x)=w451:dbl)
                n227 = Less Or Equal?(x=w451, y=w450) -> (x <= y?=w449:bool)
                n228 = Or(x=w449, y="Стоп GoTo") -> (x .or. y?=w447:bool)
                "Готово" <- w447
              }
              n229 = invoke class="AmateurStepperMotor" method="Stop"(reference=w435) -> (reference out=w433:refnum<k24>)  [unwired: 2 in, 2 out]
              n230 = property class="AmateurStepperMotor"(reference=w433) -> ("Position"=w432:dbl)  [unwired: 1 in, 2 out]
              n231 = local write "Position"(w432) -> ()
            }
          }
        }
      }
      event "set pos": Value Change {
        n232 = event-data() -> ("NewVal"=w456:bool)  [unwired: 1 in, 5 out]
        n233 = case shown="False" w456 {
          tunnel: w455 -> [_ w460]
          tunnel: "new pos" -> [_ w459]
          frame False {
          }
          frame True {
            n234 = property class="AmateurStepperMotor"(reference=w460, "Position"=w459) -> (reference out=w458:refnum<k24>)  [unwired: 1 in, 1 out]
            n235 = property class="AmateurStepperMotor"(reference=w458) -> ("Position"=w457:dbl)  [unwired: 1 in, 2 out]
            n236 = local write "Position"(w457) -> ()
          }
        }
      }
      event "Стоп": Value Change {
        n237 = event-data() -> ()  [unwired: 1 in, 6 out]
        n238 = local read "Стоп"() -> (w461:bool)
      }
    }
  }
  n239 = while {
    shift-right: [w462] -> _
    shift-left: 0 -> [w464]
    tunnel: w1 -> [_]
    stop <- w468 stop-if-true
    # "Управление Ардуино тумблерами"
    n240 = local read "Стоп"() -> (w468:bool)
    n241 = Boolean Array To Number(Boolean array="Сегменты") -> (number=w463:u32)
    n242 = Wait (ms)(milliseconds to wait=u32 10 ("millisecond timer value")) -> ()  [unwired: 1 out]
    n243 = To Long Integer(number=w463) -> (32bit integer=w462:i32)
    n244 = Not Equal?(x=w462, y=w464) -> (x != y?=w466:bool)
    n245 = case shown="True" w466 {
      tunnel: w462 -> [_ w469]
      tunnel: w464 -> [_ w470]
      frame False {
      }
      frame True {
        n246 = stacked-sequence {
          seq-local: [w473 _ _] -> [_ w478 _]
          seq-local: [w471 _ _] -> [_ w482 _]
          seq-local: [_ w483 _] -> [_ _ w520]
          tunnel: w469 -> [w475 _ _]
          tunnel: w470 -> [w474 _ _]
          frame #0 {
            # "Детектирвоание позиции и\nнаправления изменения бита"
            n247 = Subtract(x=w475, y=w474) -> (x-y=w476:i32)
            n248 = To Double Precision Float(number=w476) -> (double precision float=w477:dbl)
            n249 = Greater Than 0?(x=w476) -> (x > 0?=w473:bool)
            "+/-" <- w473
            n250 = Absolute Value(x=w477) -> (abs(x)=w472:dbl)
            n251 = Logarithm Base 2(1:w472) -> (0:w471:dbl)
            "Разряд" <- w471
          }
          frame #1 {
            # "последний включенный сегмент"
            # "Выбор бита и направления\n его измнения"
            n252 = case shown="13" w482 {
              tunnel: ["D10" "D9" "D5" "D8" "D11" "D12" "A1" "D4" "A5" "A4" "A3" "A2" "A0" "D13" "D3" "All"] -> w480
              tunnel: ["a" "b" "c" "d" "e" "f" "g" "h" "j" "k" "L" "m" "n" "p" "dp" "All"] -> w479
              frame 0, Default {
                # "a = D10"
              }
              frame 1 {
                # "b = D9"
              }
              frame 2 {
                # "c = D5"
              }
              frame 3 {
                # "d = D8"
              }
              frame 4 {
                # "e = D11"
              }
              frame 5 {
                # "f = D12"
              }
              frame 6 {
                # "g = A1"
              }
              frame 7 {
                # "h = D4"
              }
              frame 8 {
                # "j = A5"
              }
              frame 9 {
                # "k = A4"
              }
              frame 10 {
                # "L = A3"
              }
              frame 11 {
                # "m = A2"
              }
              frame 12 {
                # "n = A0"
              }
              frame 13 {
                # "p = D13"
              }
              frame 14 {
                # "dp = D3"
              }
              frame 15 {
              }
            }
            n253 = Select(t="off", s=w478, f="on") -> (s? t:f=w481:string)
            n254 = Concatenate Strings(w480, "_" ("string"), w481) -> (w483:string)
            n255 = case shown="True" w478 {
              tunnel: w479 -> [_ w487]
              frame False {
              }
              frame True {
                "Сегмент" <- w487
              }
            }
          }
          frame #2 {
            # "Передача команды в Ардуино"
            n256 = disable-structure shown="Disabled" {
              disable-tunnel: w520 -> [w522 _]
              frame Disabled {
                n257 = Equal?(x=w522, y="All_off") -> (x = y?=w525:bool)
                n258 = Equal?(x=w522, y="All_on") -> (x = y?=w523:bool)
                n259 = case shown="True" w525 {
                  frame False {
                  }
                  frame True {
                    n260 = local write "Сегменты"(bool[] [TRUE, TRUE, TRUE, TRUE, TRUE, TRUE, TRUE, TRUE, TRUE, TRUE, TRUE, TRUE, TRUE, TRUE, TRUE, TRUE] ("Сегменты")) -> ()
                  }
                }
                n261 = case shown="True" w523 {
                  frame False {
                  }
                  frame True {
                    n262 = local write "Сегменты"(bool[] [FALSE, FALSE, FALSE, FALSE, FALSE, FALSE, FALSE, FALSE, FALSE, FALSE, FALSE, FALSE, FALSE, FALSE, FALSE, FALSE] ("Сегменты")) -> ()
                  }
                }
              }
              frame Enabled {
              }
            }
            n263 = stacked-sequence {
              tunnel: w520 -> [w528 _ _]
              frame #0 {
                n264 = local write "Command"(w528) -> ()
              }
              frame #1 {
                n265 = local write "Записать"(TRUE ("Записать")) -> ()
                n266 = Wait (ms)(milliseconds to wait=u32 1000) -> ()  [unwired: 1 out]
              }
              frame #2 {
                n267 = local write "Записать"(FALSE ("Записать")) -> ()
                n268 = Wait (ms)(milliseconds to wait=u32 1000) -> ()  [unwired: 1 out]
              }
            }
          }
        }
      }
    }
  }
  n269 = call <instrlib>:"niDMM Close.vi"("error in (no error)"=w27, "instrument handle"=w28) -> ()  [unwired: 9 in, 1 out]
  n270 = while {
    tunnel: [w539] -> w29
    tunnel: w32 -> [w537]
    tunnel: w31 -> [w536]
    tunnel: [w533] -> w30
    stop <- w535 stop-if-true
    # "Настройка вольтметра NI PXI-4071"
    n271 = Wait (ms)(milliseconds to wait=u32 1) -> ()  [unwired: 1 out]
    n272 = flat-sequence {
      tunnel: [w546] -> w541
      tunnel: w537 -> [w544]
      tunnel: w536 -> [w548]
      tunnel: [w545] -> w540
      tunnel: w541 -> [w558]
      tunnel: w540 -> [w561]
      tunnel: [w557] -> w535
      tunnel: [w556] -> w533
      tunnel: [w555] -> w534
      frame #0 {
        w542 = T6 6.5 items=["3 1/2"=3.5, "4 1/2"=4.5, "5 1/2"=5.5, "6 1/2"=6.5, "7 1/2"=7.5] ("Resolution in Digits")
        n273 = Fract/Exp String To Number(string="NI DMM 1 Voltage Range 4") -> (number=w547:dbl)  [unwired: 3 in, 1 out]
        n274 = call-poly <instrlib>:"niDMM Config Measurement.vi"("Range"=w547, "Resolution in Digits"=w542, "error in (no error)"=w548, "Function"=niDMM_Function."DC Volts" ("Measurement Type"), "instrument handle"=w544) -> ("error out"=w545:errorcluster, "instrument handle out"=w546:refnum<k15>)  [unwired: 5 in]
      }
      frame #1 {
        n275 = call <instrlib>:"niDMM Read.vi"("error in (no error)"=w561, "instrument handle"=w558) -> ("error out"=w555:errorcluster, "Measurement"=w551:dbl, "instrument handle out"=w556:refnum<k15>)  [unwired: 7 in]
        n276 = Fract/Exp String To Number(string="NI DMM 1 units 4") -> (number=w559:dbl)  [unwired: 3 in, 1 out]
        n277 = Multiply(x=w559, y=w551) -> (x*y=w553:dbl)
        n278 = Absolute Value(x=w553) -> (abs(x)=→"Voltage Char" →"Voltage Char 2":dbl)
        n279 = Absolute Value(x=w553) -> (abs(x)=→"Voltage":dbl)
        n280 = Absolute Value(x=w551) -> (abs(x)=→"Voltage, V":dbl)
        n281 = local read "Стоп"() -> (w557:bool)
      }
    }
    n282 = call <vilib>:"Simple Error Handler.vi"("error in (no error)"=w534) -> ("error out"=w539:errorcluster)  [unwired: 1 in, 7 out]
  }
  n283 = invoke class="AmateurStepperMotor" method="Stop"(reference=w7) -> (reference out=w14:refnum<k24>, "Stop"=w15:refnum<k24>)  [unwired: 2 in, 1 out]
  n284 = property class="AmateurStepperMotor"(reference=w14, "HoldOn"=FALSE) -> (reference out=w13:refnum<k24>)  [unwired: 1 in, 1 out]
  n285 = invoke class="AmateurStepperMotor" method="Dispose"(reference=w13) -> (error out=w10:errorcluster)  [unwired: 2 in, 2 out]
  n286 = invoke class="SerialPort" method="Close"(reference=w20, error in=w10) -> (reference out=w9:refnum<k24>, error out=w11:errorcluster)  [unwired: 1 in, 1 out]
  n287 = invoke class="Task" method="Wait"(reference=w15) -> ()  [unwired: 2 in, 3 out]
  n288 = Close Reference(reference=w9, error in (no error)=w11) -> (error out=w12:errorcluster)
  n289 = call <vilib>:"Simple Error Handler.vi"("error in (no error)"=w12) -> ()  [unwired: 1 in, 8 out]
  n290 = VISA Close(VISA resource name=w18, error in (no error)=w17) -> (error out=w22:errorcluster)
  n291 = call <instrlib>:"niDMM Close.vi"("error in (no error)"=w29, "instrument handle"=w30) -> ()  [unwired: 9 in, 1 out]
  n292 = call <instrlib>:"niDCPower Close.vi"("instrument handle"=w34) -> ()  [unwired: 10 in, 1 out]
  n293 = call "Ophir Error Message.vi"("error in (no error)"=w22) -> ()  [unwired: 3 in, 4 out]
